vi "Stop.vi"(8 "error in (no error)":errorcluster, 11 "reference in":refnum<class "Test_Flux_Capacitor.lvclass">) -> (0 "error out":errorcluster, 3 "reference in":refnum<class "Test_Flux_Capacitor.lvclass">)   [LabVIEW 2022 SP3, in "Test_Flux_Capacitor.lvlib" / "Test_Flux_Capacitor.lvclass"]
uses:
  Test_Flux_Capacitor.lvclass
  Components/SwitchBase.lvlibp/SwitchBase.lvclass
  Components/PSU_Base.lvlibp/PSU_Base.lvclass
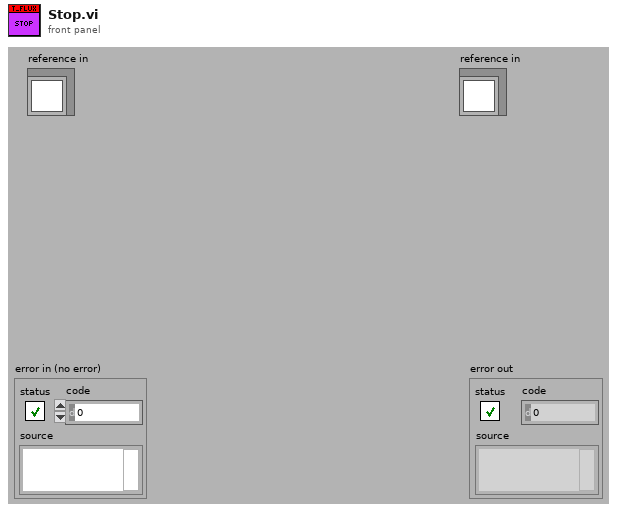
[diagram p1: front panel]
types:
  T1 = typedef "Test_Flux_Capacitor.lvlib/Test_Flux_Capacitor.lvclass/ObjectAttributes.ctl" = cluster{"Config":T2, "DMM":refnum<class "DMM_Keysight_34980A.lvclass">, "LCR":refnum<class "LCR_BK891.lvclass">, "PSU":refnum<class "PSU_Base.lvclass">, "Switch_Manager":refnum<class "SwitchBase.lvclass">, "FRAM":string, "Flux_Capacitor":refnum<class "Flux_Capacitor.lvclass">, "Frequency_Counter":refnum<class "Frequency_Counter_Base.lvclass">, "JTAG":refnum<class "JTAG_Base.lvclass">}
  T2 = typedef "Test_Flux_Capacitor.lvlib/Test_Flux_Capacitor.lvclass/Config.ctl" = cluster{"default":string}
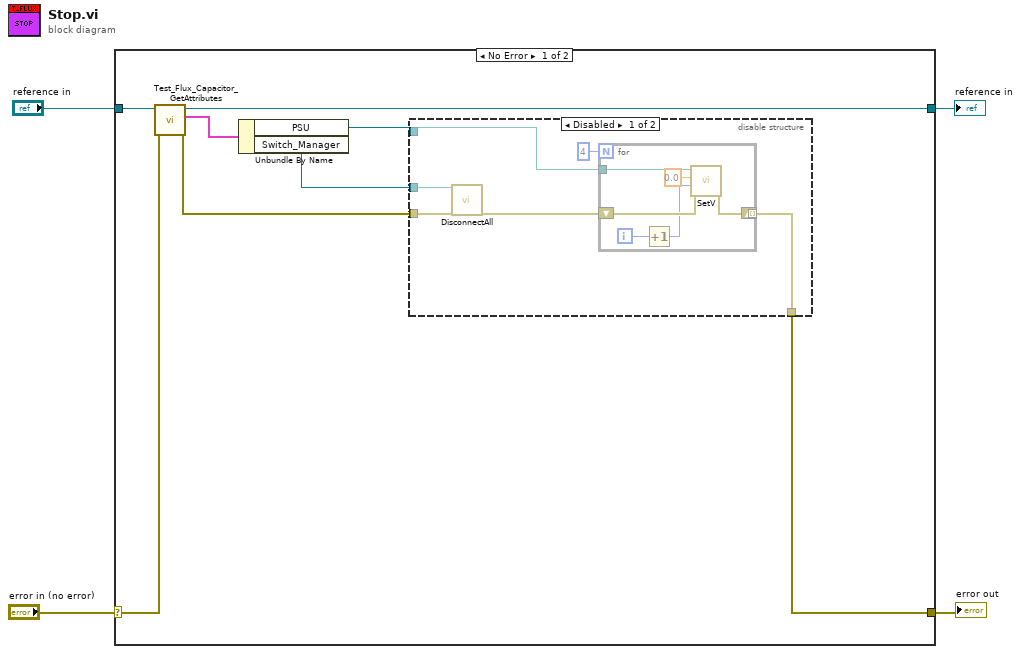
[diagram p0: block diagram]
diagram:
  n1 = case shown="No Error" "error in (no error)" {
    selector: "error in (no error)" -> [w12 w26]
    tunnel: [w5 w26] -> w3
    tunnel: [w9 w25] -> w1
    tunnel: "reference in" -> [w10 w25]
    frame No Error {
      n2 = call "Test_Flux_Capacitor_GetAttributes.vi"("error in (no error)"=w12, "reference in"=w10) -> ("error out"=w7:errorcluster, "Data"=w11:T1, "reference out"=w9:refnum<class "Test_Flux_Capacitor.lvclass">)  [unwired: 6 in, 1 out]
      n3 = Unbundle By Name(w11) -> ("PSU"=w6:refnum<class "PSU_Base.lvclass">, "Switch_Manager"=w8:refnum<class "SwitchBase.lvclass">)
      n4 = disable-structure shown="Disabled" {
        disable-tunnel: w8 -> [w18 _]
        disable-tunnel: w7 -> [w17 _]
        disable-tunnel: w6 -> [w16 _]
        disable-tunnel: [w13 _] -> w5
        frame Disabled {
          n5 = call-dynamic "DisconnectAll.vi"("reference in"=w18, "error in (no error)"=w17) -> ("error out"=w14:errorcluster)  [unwired: 16 in, 1 out]
          n6 = for {
            N: 4 -> [_]
            tunnel: w16 -> [w24]
            shift-right: [w19] -> w13
            shift-left: w14 -> [w23]
            tunnel: [w19] -> _ mode=indexing
            i -> [w22]
            n7 = Increment(x=w22) -> (x+1=w21:i32)
            n8 = call-dynamic "SetV.vi"("error in (no error)"=w23, "Chan"=w21, "V"=0.0, "reference in"=w24) -> ("error out"=w19:errorcluster)  [unwired: 6 in, 1 out]
          }
        }
        frame Enabled {
        }
      }
    }
    frame Error {
    }
  }
  "error out" <- w3
  "reference in" <- w1
